vi "Send Text using SMTP API.vi"(4 "Body":string, 5 "Carrier":enum16{"T-Mobile", "AT&T", "Verizon", "Sprint"}(ring), 6 "Subject":string, 7 "phone number":string, 10 "Password":string, 11 "Email":string) -> ()   [LabVIEW 2017]
uses:
  <vilib>/smtpClient/Set Message Text.vi
  <vilib>/smtpClient/LabVIEWSMTPClient.lvlib
panel:
  in  "TLS":bool=TRUE
  in  "Outgoing Mail Server (SMTP)":string="smtp.gmail.com"
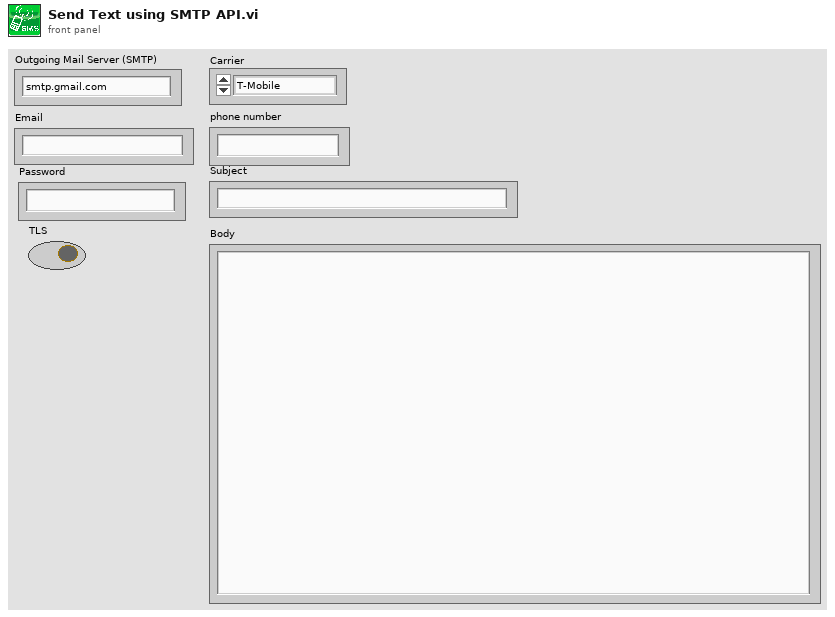
[diagram p1: front panel]
types:
  T1 = typedef "LabVIEWSMTPClient.lvlib/SmtpClientHandle.ctl" = refnum<k1>
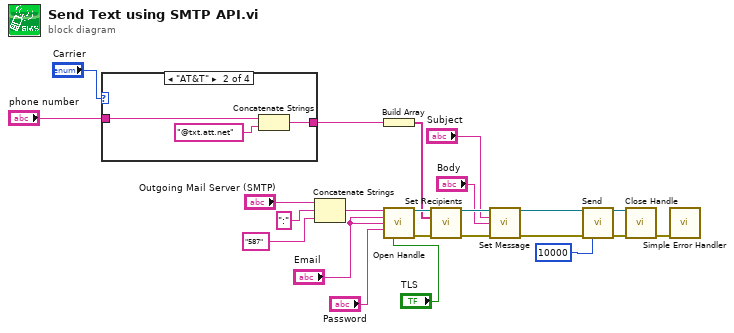
[diagram p0: block diagram]
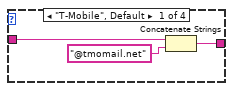
[diagram p2: hidden frame]
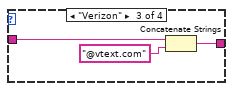
[diagram p3: hidden frame]
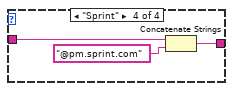
[diagram p4: hidden frame]
diagram:
  n1 = case shown="\"AT&T\"" "Carrier" {
    tunnel: "phone number" -> [w26 w28 w31 w34]
    tunnel: [w24 w29 w32 w35] -> w9
    frame "T-Mobile", Default {
      n2 = Concatenate Strings(w26, "@tmomail.net" ("string")) -> (w24:string)
    }
    frame "AT&T" {
      n3 = Concatenate Strings(w28, "@txt.att.net" ("string")) -> (w29:string)
    }
    frame "Verizon" {
      n4 = Concatenate Strings(w31, "@vtext.com" ("string")) -> (w32:string)
    }
    frame "Sprint" {
      n5 = Concatenate Strings(w34, "@pm.sprint.com") -> (w35:string)
    }
  }
  n6 = Concatenate Strings("Outgoing Mail Server (SMTP)", ":" ("string"), "587" ("Port")) -> (w4:string)
  n7 = Build Array(w9) -> (w8:string[])
  n8 = call <vilib>:"Open Handle.vi"("server address"=w4, "from"="Email", "username"="Email", "password"="Password", "use TLS (false)"="TLS") -> ("handle out"=w21:T1, "error out"=w18:errorcluster)  [unwired: 9 in]
  n9 = call <vilib>:"Set Recipients.vi"("handle in"=w21, "to"=w8, "error in (no error)"=w18) -> ("handle out"=w17:T1, "error out"=w16:errorcluster)  [unwired: 11 in]
  n10 = call-poly <vilib>:"Set Message.vi"("handle in"=w17, "subject"="Subject", "plain text message"="Body", "error in (no error)"=w16) -> ("handle out"=w13:T1, "error out"=w12:errorcluster)  [unwired: 10 in]
  n11 = call <vilib>:"Send.vi"("handle in"=w13, "error in (no error)"=w12, "timeout in ms (10000)"=10000) -> ("handle out"=w11:T1, "error out"=w10:errorcluster)  [unwired: 10 in, 1 out]
  n12 = call <vilib>:"Close Handle.vi"("handle in"=w11, "error in (no error)"=w10) -> ("error out"=w1:errorcluster)  [unwired: 12 in, 1 out]
  n13 = call <vilib>:"Simple Error Handler.vi"("error in (no error)"=w1) -> ()  [unwired: 4 in, 5 out]
